vi "Set DSSS Data Rate (Mbps).vi"(8 "error in (no error)":errorcluster, 10 "DSSS Data Rate (Mbps)":T1, 11 "niDTS WLAN Dut in":refnum<class "niDTS WLAN Dut.lvclass">) -> (0 "error out":errorcluster, 3 "niDTS WLAN Dut out":refnum<class "niDTS WLAN Dut.lvclass">)   [LabVIEW 2015, in "niDTS WLAN.lvlib" / "niDTS WLAN Dut.lvclass"]
doc: "Sets the data rate for the DSSS Standard (802.11b).\n\nCallbacks:\n* Update Type\n* Update Payload Length"
uses:
  niDTS WLAN Dut.lvclass
  Includes/niDTS WLAN INC DSSS Data Rate.ctl
  niDTS WLAN Dut.lvclass/niDTS WLAN Dut.ctl
  niDTS WLAN.lvlib
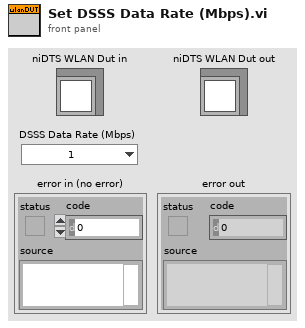
[diagram p1: front panel]
types:
  T1 = typedef "niDTS WLAN.lvlib/niDTS WLAN INC DSSS Data Rate.ctl" = enum16{"1", "2", "5.5", "11"}
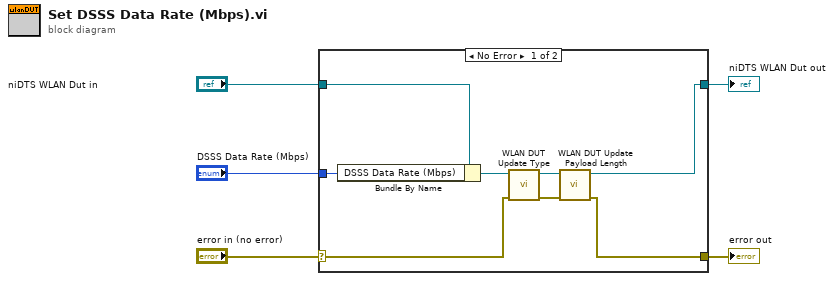
[diagram p0: block diagram]
diagram:
  n1 = case shown="No Error" "error in (no error)" {
    selector: "error in (no error)" -> [w8 w14]
    tunnel: [w7 w14] -> w4
    tunnel: [w6 w15] -> w2
    tunnel: "niDTS WLAN Dut in" -> [w13 w15]
    tunnel: "DSSS Data Rate (Mbps)" -> [w12 _]
    frame No Error {
      n2 = Bundle By Name(cluster=w13, "DSSS Data Rate (Mbps)"=w12) -> (w9:refnum<class "niDTS WLAN Dut.lvclass">)
      n3 = call-dynamic "WLAN DUT Update Type.vi"("error in (no error)"=w8, "niDTS WLAN DUT in"=w9) -> ("error out"=w11:errorcluster, "niDTS WLAN DUT out"=w10:refnum<class "niDTS WLAN Dut.lvclass">)  [unwired: 8 in]
      n4 = call-dynamic "WLAN DUT Update Payload Length.vi"("error in (no error)"=w11, "niDTS WLAN DUT in"=w10) -> ("error out"=w7:errorcluster, "niDTS WLAN DUT out"=w6:refnum<class "niDTS WLAN Dut.lvclass">)  [unwired: 8 in]
    }
    frame Error {
    }
  }
  "error out" <- w4
  "niDTS WLAN Dut out" <- w2
